vi "receive message.vi"(8 "error in (no error)":errorcluster, 11 "Server in":refnum<class "Server.lvclass">) -> (0 "error out":errorcluster, 3 "Server out":refnum<class "Server.lvclass">)   [LabVIEW 2018, in "Server.lvclass"]
uses:
  Server.lvclass
  Server.lvclass/Server.ctl
  RxTx/RxTx.lvclass
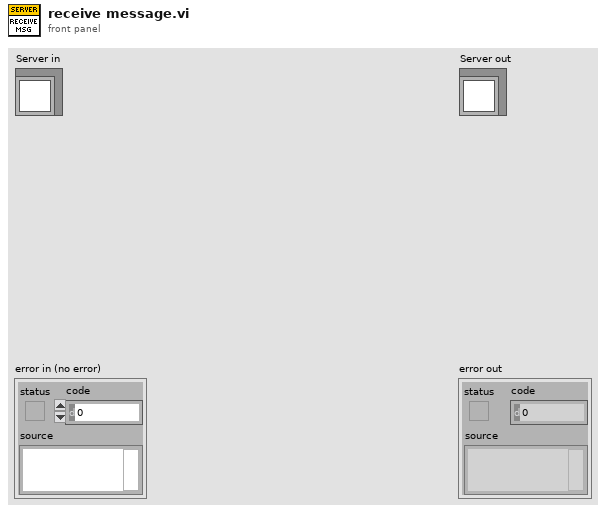
[diagram p1: front panel]
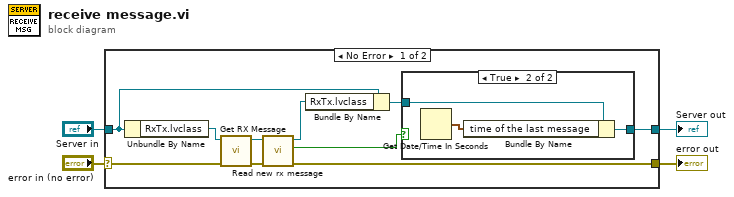
[diagram p0: block diagram]
diagram:
  n1 = case shown="No Error" "error in (no error)" {
    selector: "error in (no error)" -> [w13 w20]
    tunnel: [w6 w20] -> w3
    tunnel: [w12 w19] -> w1
    tunnel: "Server in" -> [w11 w19]
    frame No Error {
      n2 = Unbundle By Name(w11) -> ("RxTx.lvclass"=w14:refnum<class "RxTx.lvclass">)
      n3 = call "Get RX Message.vi"("error in (no error)"=w13, "RxTx in"=w14) -> ("error out"=w7:errorcluster, "RxTx out"=w9:refnum<class "RxTx.lvclass">)  [unwired: 8 in]
      n4 = call-dynamic "Read new rx message.vi"("error in (no error)"=w7, "RxTx in"=w9) -> ("error out"=w6:errorcluster, "new rx message"=w5:bool, "RxTx out"=w8:refnum<class "RxTx.lvclass">)  [unwired: 7 in]
      n5 = Bundle By Name(cluster=w11, "RxTx.lvclass"=w8) -> (w10:refnum<class "Server.lvclass">)
      n6 = case shown="True" w5 {
        tunnel: w10 -> [w15 w18]
        tunnel: [w15 w17] -> w12
        frame False {
        }
        frame True {
          n7 = Get Date/Time In Seconds() -> (seconds since 1Jan1904=w16:timestamp)
          n8 = Bundle By Name(cluster=w18, "time of the last message"=w16) -> (w17:refnum<class "Server.lvclass">)
        }
      }
    }
    frame Error {
    }
  }
  "error out" <- w3
  "Server out" <- w1
